vi "format set border color.vi"(8 "error in (no error)":errorcluster, 10 "color":u32, 11 "format":u32) -> (0 "error out":errorcluster)   [LabVIEW 8.6]
doc: "void format_set_border_color(lxw_format format, lxw_color_t color);"
uses:
  pending_lvxlsxwriter/xlsxwriter.dll
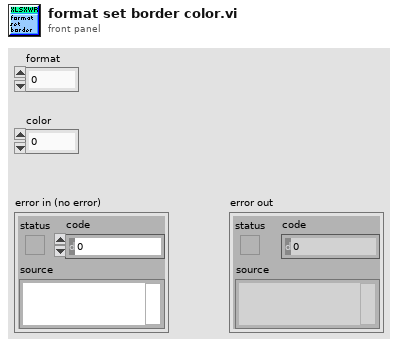
[diagram p1: front panel]
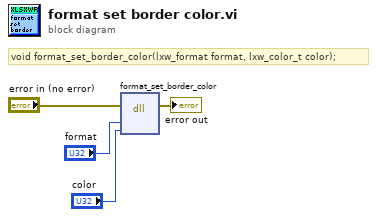
[diagram p0: block diagram]
diagram:
  # "void format_set_border_color(lxw_format format, lxw_color_t color);"
  n1 = dll-call lib="C:/Users/WDAGUtilityAccount/Desktop/pending_lvxlsxwriter/xlsxwriter.*" fn="format_set_border_color"(error in="error in (no error)", "format"="format", "color"="color") -> (error out=→"error out":errorcluster)  [unwired: 5 in, 1 out]
